vi "GetImage.vi"(8 "error in (no error)":errorcluster, 11 "GEECS_Image in":refnum<class "GEECS_Image.lvclass">) -> (0 "error out":errorcluster, 1 "Image received":bool, 2 "Image Out":T1, 3 "GEECS_Image out":refnum<class "GEECS_Image.lvclass">)   [LabVIEW 2020, in "GEECS_Image.lvclass"]
uses:
  GEECS_Image.lvclass
  <vilib>/vision/Image Controls.llb/IMAQ Image.ctl
  GEECS_Image.lvclass/GEECS_Image.ctl
panel:
  out "OK":bool[](array[boolean])
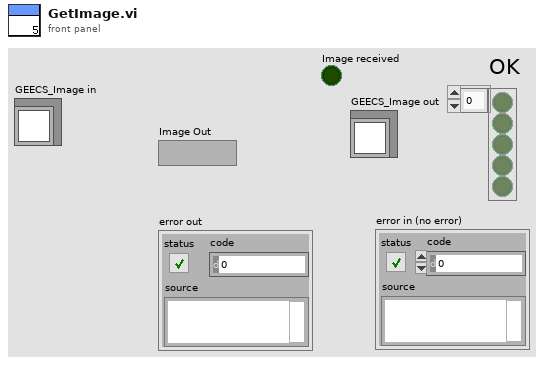
[diagram p1: front panel]
types:
  T1 = typedef "IMAQ Image.ctl" = refnum<image>
  T2 = typedef "SubscriberCluster_TypDEf.ctl" = cluster{"tcp data event":T3, "Event Registration Refnum":refnum<event-registration>, "data queue":refnum<queue>, "Devices":string[], "Alias":string[], "Variable header":string[], "Devices ALL":string[]}
  T3 = typedef "tcp_new_data_event.ctl" = refnum<user-event>
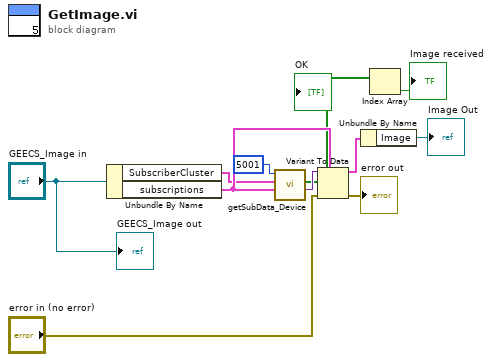
[diagram p0: block diagram]
diagram:
  n1 = Unbundle By Name("GEECS_Image in") -> ("SubscriberCluster"=w7:T2, "subscriptions"=w8:cluster{"Image":T1})
  n2 = call "getSubData_Device.vi"("variant in"=w8, "SubscriberCluster"=w7, "timeout"=5001) -> ("variant out"=w6:variant, "OK"=w2:bool[])  [unwired: 4 in, 3 out]
  "OK" <- w2
  n3 = Variant To Data(error in="error in (no error)", type=w8, Variant=w6) -> (data=w10:cluster{"Image":T1}, error out=→"error out":errorcluster)
  n4 = Unbundle By Name(w10) -> ("Image"=→"Image Out":T1)
  n5 = Index Array(array=w2) -> (element=→"Image received":bool)  [unwired: 1 in]
  "GEECS_Image out" <- "GEECS_Image in"
